vi "Reset ChipKit.vi"(8 "Error In":errorcluster, 11 "VISA resource":refnum<visa-resource-name>) -> (0 "Error Out":errorcluster, 3 "VISA resource":refnum<visa-resource-name>)   [LabVIEW 2011, in "LabVIEW Interface for ChipKit.lvlib"]
uses:
  LabVIEW Interface for ChipKit.lvlib
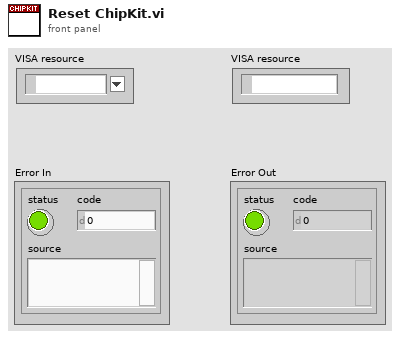
[diagram p1: front panel]
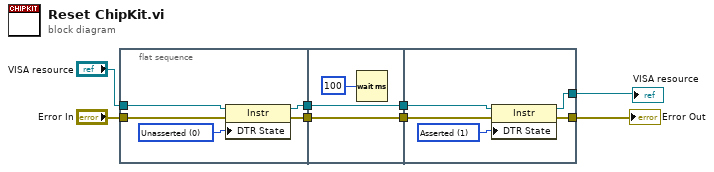
[diagram p0: block diagram]
diagram:
  n1 = flat-sequence {
    tunnel: "Error In" -> [w13]
    tunnel: "VISA resource" -> [w12]
    tunnel: [w11] -> w8
    tunnel: [w10] -> w7
    tunnel: [w16] -> w6
    tunnel: w8 -> [w16]
    tunnel: [w15] -> w5
    tunnel: w7 -> [w15]
    tunnel: w6 -> [w21]
    tunnel: [w20] -> w1
    tunnel: w5 -> [w19]
    tunnel: [w18] -> w3
    frame #0 {
      w9 = i16 0 items=["Unknown"=-1, "Unasserted"=0, "Asserted"=1] ("Serial Settings:Modem Line Settings:Line DTR State")
      n2 = property class="Instr"(reference=w12, error in=w13, "DTR State"=w9) -> (reference out=w11:refnum<visa-resource-name>, error out=w10:errorcluster)
    }
    frame #1 {
      n3 = Wait (ms)(milliseconds to wait=u32 100) -> ()  [unwired: 1 out]
    }
    frame #2 {
      w17 = i16 1 items=["Unknown"=-1, "Unasserted"=0, "Asserted"=1] ("Serial Settings:Modem Line Settings:Line DTR State")
      n4 = property class="Instr"(reference=w21, error in=w19, "DTR State"=w17) -> (reference out=w20:refnum<visa-resource-name>, error out=w18:errorcluster)
    }
  }
  "Error Out" <- w3
  "VISA resource" <- w1
